vi "Leaf.vi"() -> ()   [LabVIEW 2012]
uses:
  Global_Telescopio.vi
panel:
  in  "ok":bool
  in  "Senha:":string
  out "String":string="\n\n\nATENÇÃO: Nível Crítico de Umidade\nEntre em contato com o assistente noturno."
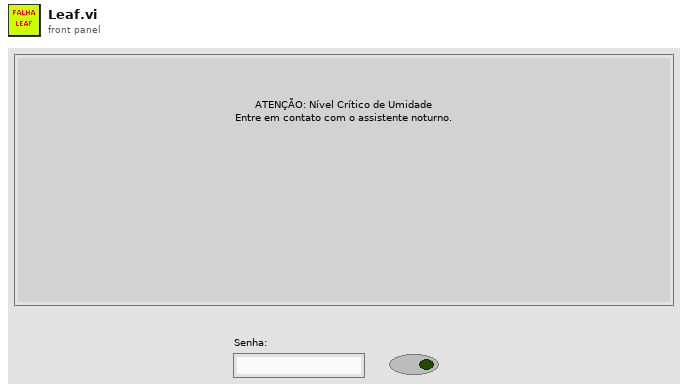
[diagram p1: front panel]
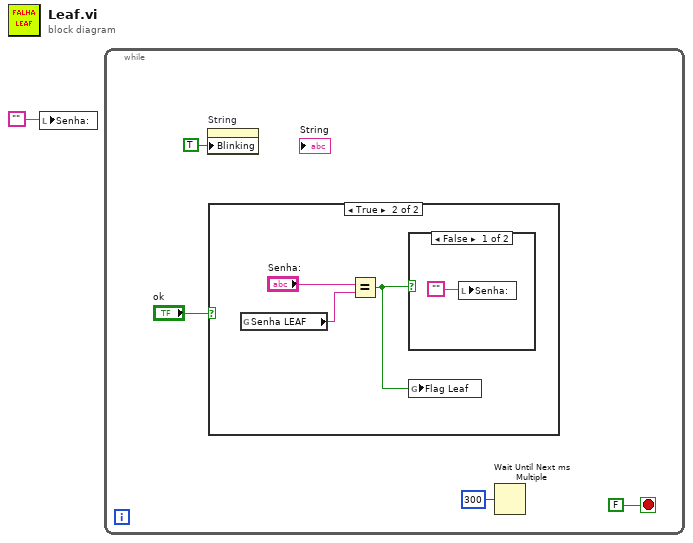
[diagram p0: block diagram]
diagram:
  n1 = local write "Senha:"("") -> ()
  n2 = while {
    stop <- FALSE stop-if-true
    n3 = property on="String" class="Str"("Blinking"=TRUE) -> ()  [unwired: 2 in, 2 out]
    n4 = case shown="True" "ok" {
      frame False {
      }
      frame True {
        n5 = global read "Global_Telescopio.vi" "Senha LEAF"() -> (w7:string)
        n6 = Equal?(x="Senha:", y=w7) -> (x = y?=w6:bool)
        n7 = case shown="False" w6 {
          frame False {
            n8 = local write "Senha:"("") -> ()
          }
          frame True {
          }
        }
        n9 = global write "Global_Telescopio.vi" "Flag Leaf"(w6) -> ()
      }
    }
    n10 = Wait Until Next ms Multiple(millisecond multiple=u32 300) -> ()  [unwired: 1 out]
  }
